vi "SubVI_Edge_element_Auto.vi"(8 "Error In":errorcluster, 9 "Auto":bool, 10 "Parameter_Edge":T3={"ROI Descriptor"={"Global Rectangle"=[], "Contours"=[]}, "Edge Options"={"Edge Polarity"=0, "Kernel Size"=3, "Width"=3, "Minimum Edge Strength"=10.0, "Interpolation Type"=enum."Bilinear Fixed", "Data Processing Method"=enum."Average"}, "Scan Direction"=0, "Step Size"=5} {"Edge Options"."Edge Polarity" items=["All Edges", "Rising Edges", "Falling Edges"]; "Edge Options"."Minimum Edge Strength" format="%.2f"; "Edge Options"."Width" step=2; "Edge Options"."Kernel Size" step=2; "Scan Direction" items=["Left To Right", "Right To Left", "Top To Bottom", "Bottom To Top"]; "ROI Descriptor"."Contours"."Type" items=["No Selection", "Point", "Line", "Rectangle", "Oval", "Polygon", "Free", "Annulus", "Unused2", "Unused3", "Broken Line", "Free Hand Line", "Rotated Rectangle"]}, 11 "Image In":T4) -> (0 "Error Out":errorcluster, 2 "Location":cluster{"X":sgl, "Y":sgl}[](array[cluster]) {"Y" format="%.2g"; "X" format="%.2f"}, 3 "Image Out":T4)   [LabVIEW 2013]
uses:
  <vilib>/vision/Image Controls.llb/IMAQ Image.ctl
  <vilib>/vision/Measure.llb/Edge Options.ctl
  <vilib>/vision/Measure.llb/Edge Polarity.ctl
  <vilib>/vision/NI_Vision_Development_Module.lvlib
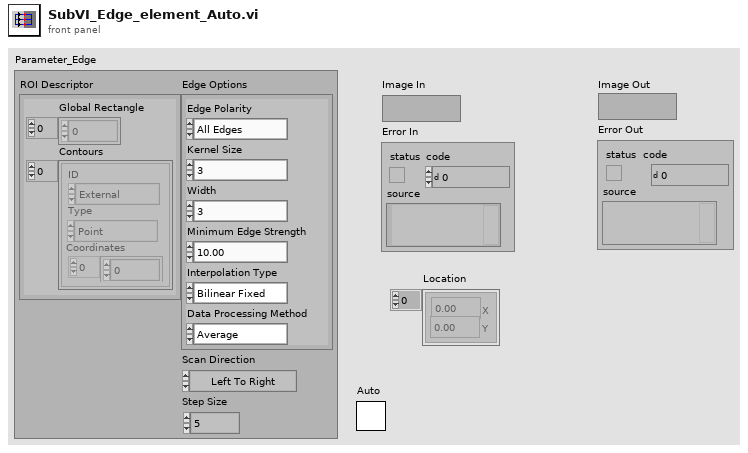
[diagram p1: front panel]
types:
  T1 = typedef "Edge Options.ctl" = cluster{"Edge Polarity":T2, "Kernel Size":u32, "Width":u32, "Minimum Edge Strength":sgl, "Interpolation Type":enum32{"Zero Order", "Bilinear", "Quadratic", "Cubic", "Bilinear Fixed"}, "Data Processing Method":enum32{"Average", "Median"}}
  T2 = typedef "Edge Polarity.ctl" = u32
  T3 = cluster{"ROI Descriptor":cluster{"Global Rectangle":i32[], "Contours":cluster{"ID":enum32{"External", "Internal"}, "Type":u32, "Coordinates":i32[]}[]}, "Edge Options":T1, "Scan Direction":u16, "Step Size":u32}
  T4 = typedef "IMAQ Image.ctl" = refnum<image>
  T5 = enum16{"Get First Edge", "Get First + Last Edge", "Get All Edges", "Get Best Edge"}
  T6 = cluster{"ID":enum32{"External", "Internal"}, "Type":u32, "Coordinates":i32[]}
  T7 = typedef "ROI Descriptor" = cluster{"Global Rectangle":i32[], "Contours":cluster{"ID":enum32{"External", "Internal"}, "Type":u32, "Coordinates":i32[]}[]}
  T8 = cluster{"Global Rectangle":i32[], "Contours":cluster{"ID":enum32{"External", "Internal"}, "Type":u32, "Coordinates":i32[]}[]}
  T9 = typedef "Search Line.ctl" = cluster{"Start Point":cluster{"X":sgl, "Y":sgl}, "End Point":cluster{"X":sgl, "Y":sgl}, "Edge Info":T10[], "Edge Map":dbl[], "Calibration Valid":bool}
  T10 = typedef "Edge New.ctl" = cluster{"Location (Pixel)":cluster{"X":sgl, "Y":sgl}, "Location (Real-World)":cluster{"X":sgl, "Y":sgl}, "Distance (Pixel)":dbl, "Distance (Real-World)":dbl, "Strength":dbl, "Noise":dbl, "Rising?":bool}
  T11 = cluster{"ID":enum32{"External", "Internal"}, "Type":u32, "Coordinates":i32[]}[]
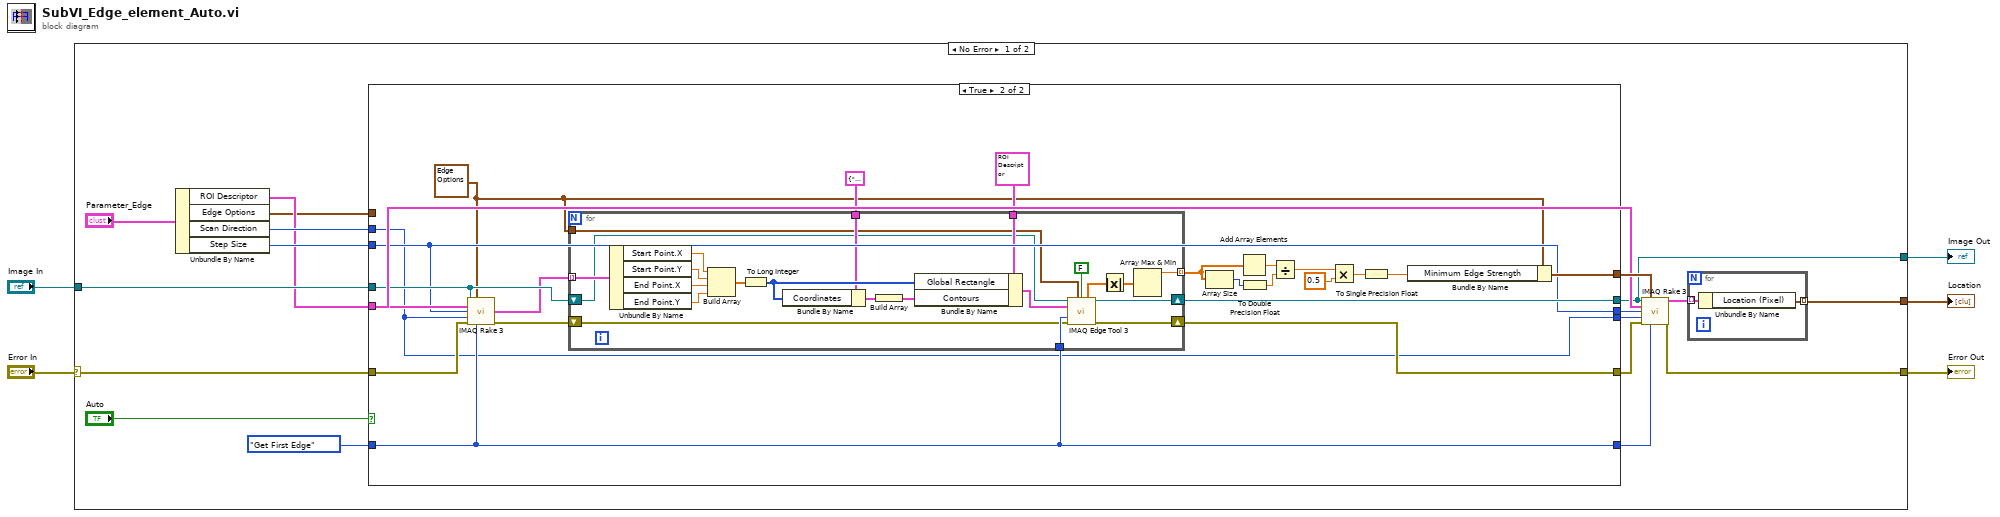
[diagram p0: block diagram]
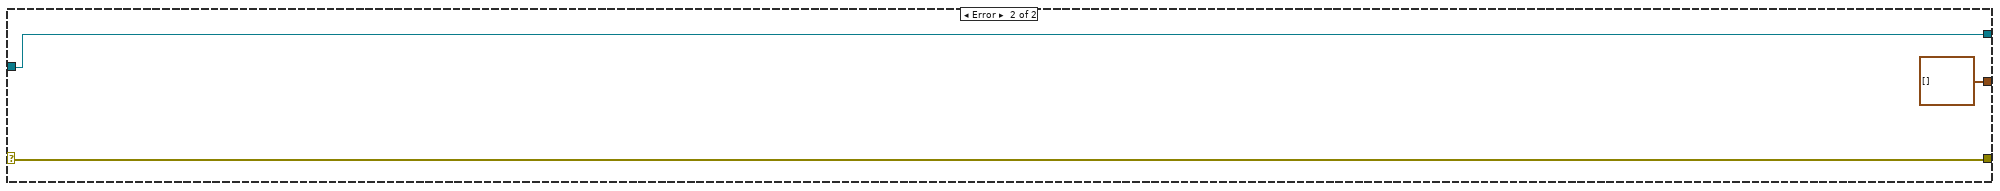
[diagram p3: hidden frame]
diagram:
  n1 = case shown="No Error" "Error In" {
    selector: "Error In" -> [w10 w77]
    tunnel: "Image In" -> [w23 w78]
    tunnel: [w9 w77] -> w3
    tunnel: [w8 w78] -> w2
    tunnel: [w7 cluster{"X":sgl, "Y":sgl}[] []] -> w1
    frame No Error {
      n2 = Unbundle By Name("Parameter_Edge") -> ("ROI Descriptor"=w12:T8, "Edge Options"=w11:T1, "Scan Direction"=w13:u16, "Step Size"=w14:u32)
      n3 = case shown="True" "Auto" {
        tunnel: w12 -> [_ w53]
        tunnel: w10 -> [w30 w52]
        tunnel: w23 -> [w31 w51]
        tunnel: [w31 w50] -> w8
        tunnel: [w26 w33] -> w22
        tunnel: [w27 w34] -> w21
        tunnel: [w28 w39] -> w20
        tunnel: [w29 w35] -> w19
        tunnel: [w30 w37] -> w18
        tunnel: T5."Get First Edge" ("Process") -> [w29 w35]
        tunnel: w11 -> [w28 _]
        tunnel: w13 -> [w26 w33]
        tunnel: w14 -> [w27 w34]
        frame False {
        }
        frame True {
          w32 = T1 {"Edge Polarity"=0, "Kernel Size"=3, "Width"=3, "Minimum Edge Strength"=10.0, "Interpolation Type"=enum."Bilinear Fixed", "Data Processing Method"=enum."Average"} ("Edge Options")
          n4 = call "IMAQ Rake 3"("Image"=w51, "Edge Options"=w32, "ROI Descriptor"=w53, "Step Size"=w34, "Scan Direction"=w33, "error in (no error)"=w52, "Process"=w35) -> ("Search Lines"=w49:T9[], "error out"=w38:errorcluster)  [unwired: 5 in, 2 out]
          n5 = for {
            tunnel: w49 -> [w75] mode=indexing
            tunnel: w35 -> [w67]
            tunnel: T7 {"Global Rectangle"=[0, 0, 0, 0], "Contours"=[{"ID"=enum."External", "Type"=2, "Coordinates"=[0, 0, 0, 0]}]} ("ROI Descriptor") -> [w65]
            tunnel: T6 {"ID"=enum."External", "Type"=2, "Coordinates"=[0, 0, 0, 0]} -> [w66]
            tunnel: w32 -> [w64]
            shift-right: [w57] -> w50
            shift-left: w51 -> [w56]
            tunnel: [w63] -> w36 mode=indexing
            shift-right: [w54] -> w37
            shift-left: w38 -> [w55]
            n6 = Unbundle By Name(w75) -> ("Start Point.X"=w74:sgl, "Start Point.Y"=w73:sgl, "End Point.X"=w72:sgl, "End Point.Y"=w71:sgl)
            n7 = Build Array(w74, w73, w72, w71) -> (w70:sgl[])
            n8 = To Long Integer(number=w70) -> (32bit integer=w68:i32[])
            n9 = Bundle By Name(cluster=w66, "Coordinates"=w68) -> (w69:T6)
            n10 = Build Array(w69) -> (w61:T11)
            n11 = Bundle By Name(cluster=w65, "Global Rectangle"=w68, "Contours"=w61) -> (w60:T7)
            n12 = call "IMAQ Edge Tool 3"("Image"=w56, "Edge Options"=w64, "Optimized Mode"=FALSE, "ROI Descriptor"=w60, "Process"=w67, "error in (no error)"=w55) -> ("Image (duplicate)"=w57:T4, "Gradient Values"=w58:dbl[], "error out"=w54:errorcluster)  [unwired: 5 in, 2 out]
            n13 = Absolute Value(x=w58) -> (abs(x)=w59:dbl[])
            n14 = Array Max & Min(array=w59) -> (max value=w63:dbl)  [unwired: 3 out]
          }
          n15 = Array Size(array=w36) -> (size(s)=w42:i32)
          n16 = Add Array Elements(numeric array=w36) -> (sum=w47:dbl)
          n17 = To Double Precision Float(number=w42) -> (double precision float=w46:dbl)
          n18 = Divide(x=w47, y=w46) -> (x/y=w45:dbl)
          n19 = Multiply(x=w45, y=0.5) -> (x*y=w41:dbl)
          n20 = To Single Precision Float(number=w41) -> (single precision float=w40:sgl)
          n21 = Bundle By Name(cluster=w32, "Minimum Edge Strength"=w40) -> (w39:T1)
        }
      }
      n22 = call "IMAQ Rake 3"("Image"=w8, "Edge Options"=w20, "ROI Descriptor"=w12, "Step Size"=w21, "Scan Direction"=w22, "error in (no error)"=w18, "Process"=w19) -> ("First Edges"=w17:T10[], "error out"=w9:errorcluster)  [unwired: 5 in, 2 out]
      n23 = for {
        tunnel: w17 -> [w25] mode=indexing
        tunnel: [w24] -> w7 mode=indexing
        n24 = Unbundle By Name(w25) -> ("Location (Pixel)"=w24:cluster{"X":sgl, "Y":sgl})
      }
    }
    frame Error {
    }
  }
  "Error Out" <- w3
  "Image Out" <- w2
  "Location" <- w1
